vi "Do Request.vi"(7 "Processing In":refnum<class "Processing.lvclass">, 11 "File Upload Controller in":refnum<class "File Upload Controller.lvclass">) -> (0 "error out":errorcluster, 5 "Processing":refnum<class "Processing.lvclass">)   [LabVIEW 2020, in "File Upload Controller.lvclass"]
uses:
  File Upload Controller.lvclass
  lv-http-util/HTTP Utils/Request/Request.lvclass
  lv-http-util/HTTP Utils/FormField/FormField.lvclass
  lv-http-util/HTTP Utils/Response/Response.lvclass
  lv-http-server/HTTP Server/Processing/Processing.lvclass
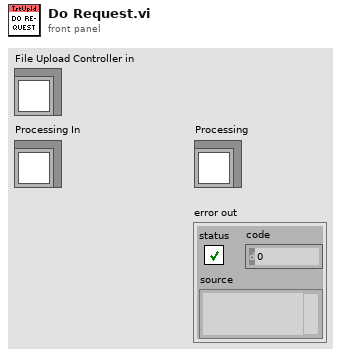
[diagram p1: front panel]
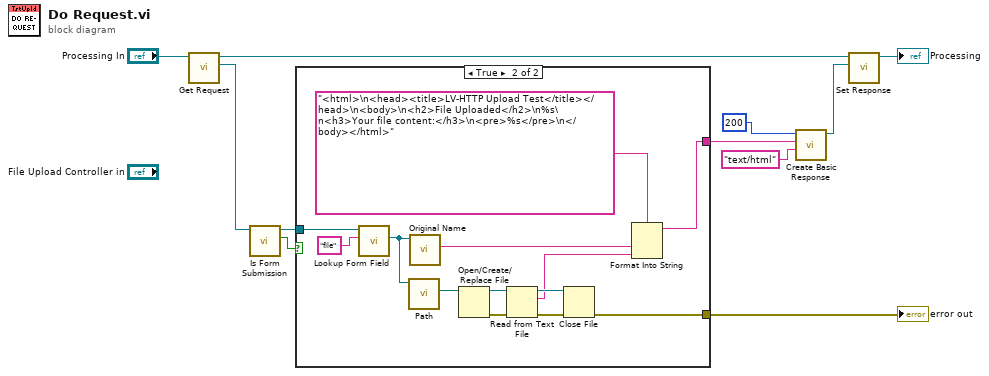
[diagram p0: block diagram]
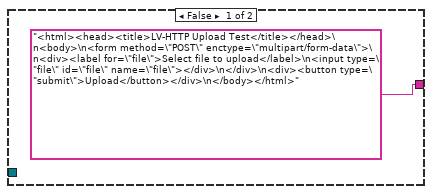
[diagram p2: hidden frame]
diagram:
  n1 = call "Get Request.vi"("Processing in"="Processing In") -> ("Request"=w11:refnum<class "Request.lvclass">, "Processing out"=w3:refnum<class "Processing.lvclass">)  [unwired: 9 in]
  n2 = call "Is Form Submission.vi"("Request in"=w11) -> ("Is Form Submission?"=w10:bool, "Request out"=w9:refnum<class "Request.lvclass">)  [unwired: 8 in, 1 out]
  n3 = case shown="True" w10 {
    tunnel: w9 -> [_ w25]
    tunnel: [_ w17] -> w8
    tunnel: ["<html><head><title>LV-HTTP Upload Test</title></head>\n<body>\n<form method=\"POST\" enctype=\"multipart/form-data\">\n<div><label for=\"file\">Select file to upload</label>\n<input type=\"file\" id=\"file\" name=\"file\"></div>\n</div>\n<div><button type=\"submit\">Upload</button></div>\n</body></html>" w13] -> w7
    frame False {
    }
    frame True {
      n4 = call "Lookup Form Field.vi"("Name"="file", "Request in"=w25) -> ("Field"=w23:refnum<class "FormField.lvclass">)  [unwired: 6 in, 3 out]
      n5 = call "Path.vi"("FormField in"=w23) -> ("Path"=w22:path)  [unwired: 8 in, 2 out]
      n6 = call "Original Name.vi"("FormField in"=w23) -> ("Original Name"=w15:string)  [unwired: 8 in, 2 out]
      n7 = Open/Create/Replace File(file path (use dialog)=w22) -> (refnum out=w21:refnum<file>, error out=w20:errorcluster)  [unwired: 5 in, 1 out]
      n8 = Read from Text File(file (use dialog)=w21, error in=w20) -> (refnum out=w18:refnum<file>, text=w14:string, error out=w19:errorcluster)  [unwired: 2 in, 1 out]
      n9 = Close File(refnum=w18, error in=w19) -> (error out=w17:errorcluster)  [unwired: 1 out]
      n10 = Format Into String(format string="<html>\n<head><title>LV-HTTP Upload Test</title></head>\n<body>\n<h2>File Uploaded</h2>\n%s\n<h3>Your file content:</h3>\n<pre>%s</pre>\n</body></html>", w15, w14) -> (resulting string=w13:string)  [unwired: 2 in, 1 out]
    }
  }
  "error out" <- w8
  n11 = call "Create Basic Response.vi"("Content-Type (text/plain)"="text/html", "Payload"=w7, "Status Code"=u16 200) -> ("Response out"=w1:refnum<class "Response.lvclass">)  [unwired: 7 in, 1 out]
  n12 = call "Set Response.vi"("Response"=w1, "Processing in"=w3) -> ("Processing out"=→"Processing":refnum<class "Processing.lvclass">)  [unwired: 9 in]
